vi "UpdateCamera.vi"(8 "error in (no error)":errorcluster, 11 "Control Window in":refnum<class "Control Window.lvclass">) -> (0 "error out":errorcluster, 3 "Control Window out":refnum<class "Control Window.lvclass">)   [LabVIEW 2015, in "Control Window.lvclass"]
uses:
  Control Window.lvclass
  Control Window.lvclass/Control Window.ctl
  3D Scene/3D Scene.lvclass
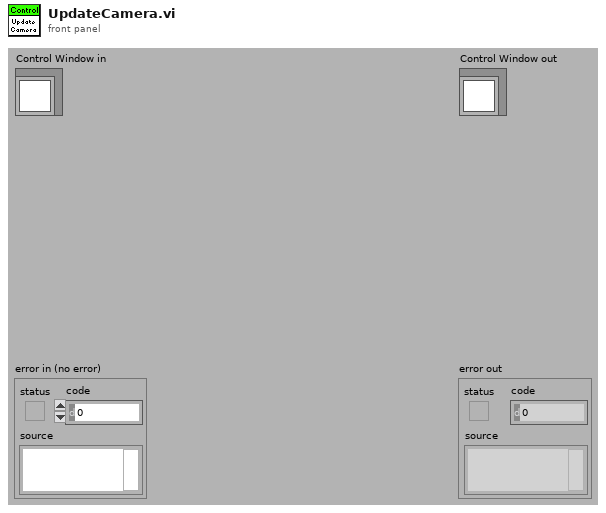
[diagram p1: front panel]
types:
  T1 = typedef "3D Point.ctl" = cluster{"X":sgl, "Y":sgl, "Z":sgl}
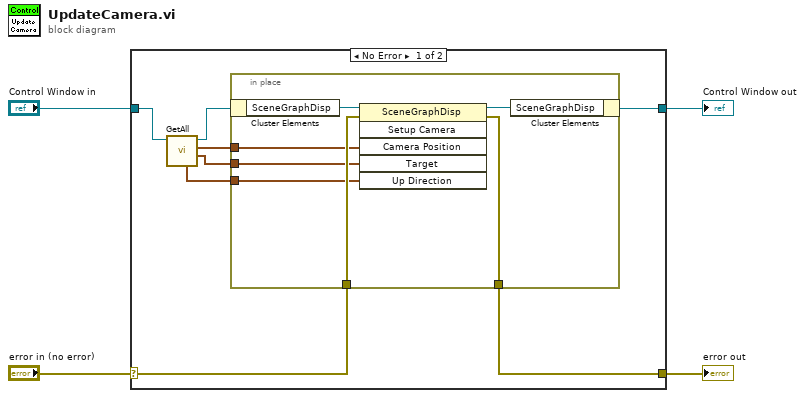
[diagram p0: block diagram]
diagram:
  n1 = case shown="No Error" "error in (no error)" {
    selector: "error in (no error)" -> [w10 w21]
    tunnel: [w11 w21] -> w3
    tunnel: "Control Window in" -> [w6 w20]
    tunnel: [w12 w20] -> w2
    frame No Error {
      n2 = call "GetAll.vi"("3D Scene in"=w6) -> ("Target"=w8:T1, "Position"=w9:T1, "3D Scene out"=w5:refnum<class "Control Window.lvclass">, "Up"=w7:T1)  [unwired: 6 in, 1 out]
      n3 = in-place {
        in-place-border: [w17] -> w11
        in-place-border: w10 -> [w16]
        in-place-border: w9 -> [w15]
        in-place-border: w8 -> [w14]
        in-place-border: w7 -> [w13]
        n4 = in-place-cluster #1(w5) -> ("SceneGraphDisp"=w19:refnum<vi>)
        n5 = invoke class="SceneGraphDisp" method="Setup Camera"(reference=w19, error in=w16, "Camera Position"=w15, "Target"=w14, "Up Direction"=w13) -> (reference out=w18:refnum<vi>, error out=w17:errorcluster)  [unwired: 1 in, 4 out]
        n6 = in-place-cluster #1("SceneGraphDisp"=w18) -> (w12:refnum<class "Control Window.lvclass">)
      }
    }
    frame Error {
    }
  }
  "error out" <- w3
  "Control Window out" <- w2
